vi "Create.vi"(5 "IsEqual In":refnum<class "IsEqual.lvclass">, 8 "error in (no error)":errorcluster, 10 "Expected":variant) -> (0 "error out":errorcluster, 3 "IsEqual":refnum<class "IsEqual.lvclass">)   [LabVIEW 2017, in "Transparent Assertions.lvlib" / "Constraints.lvlib" / "IsEqual.lvclass"]
uses:
  IsEqual.lvclass
  IsEqual.lvclass/IsEqual.ctl
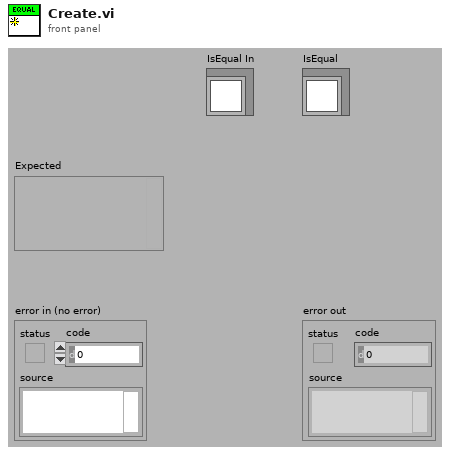
[diagram p1: front panel]
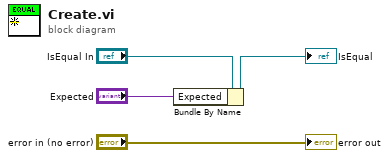
[diagram p0: block diagram]
diagram:
  n1 = Bundle By Name(cluster="IsEqual In", "Expected"="Expected") -> (→"IsEqual":refnum<class "IsEqual.lvclass">)
  "error out" <- "error in (no error)"
